vi "Check Channel Technique Compatibility.vi"(8 "error in (no error)":errorcluster, 9 "Technique in":T1, 10 "Channel":u8, 11 "Potentiostat Galvanostat in":refnum<class "Potentiostat Galvanostat.lvclass">) -> (0 "error out":errorcluster, 1 "Technique out":T1, 2 "Is Comapatible?":bool, 3 "Potentiostat Galvanostat out":refnum<class "Potentiostat Galvanostat.lvclass">)   [LabVIEW 2018, in "Potentiostat Galvanostat.lvclass"]
uses:
  Potentiostat Galvanostat.lvclass
  Controls/Technique List.ctl
  Controls/Error Codes.ctl
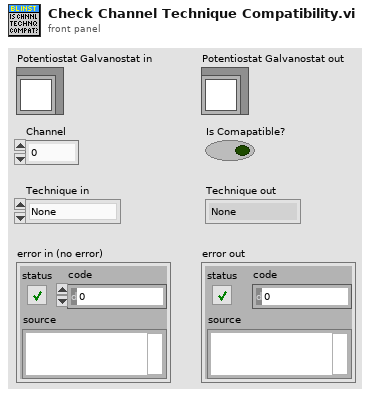
[diagram p1: front panel]
types:
  T1 = typedef "Potentiostat Galvanostat.lvclass/Technique List.ctl" = enum16{"None", "ocv", "cv", "biovscan", "ca", "cp", "iscan", "vscan", "lasv", "load", "pow", "peis", "geis", "seisp", "seisg", "dpv", "swv", "npv", "mpv", "dnpv", "dpa", "evt", "lp", "gc", "cpp", "pdp", "psp", "zra", "ircmp", "pzir", "gzir", "loop", "TO", "TI", "TOS", "vscanlimit", "iscanlimit", "mp", "casp", "casg", "calimit", "cplimit"}
  T2 = typedef "Potentiostat Galvanostat.lvclass/Error Codes.ctl" = i32
  T3 = typedef "Potentiostat Galvanostat.lvclass/Channel Information.ctl" = cluster{"Channel":i32, "Board Version":i32, "Board Serial Number":i32, "Firmware Code":T4, "Firmware Version":i32, "Xilinx Version":i32, "Amplifier Code":T5, "Number of Amplifiers":i32, "Low Current Board Present?":i32, "Impedance Capable?":i32, "RESERVED":i32, "RESERVED 2":i32, "Memory Size":i32, "Memory Filled (in Bytes)":i32, "Channel State":T6, "Maximum Current Range Allowed":T7, "Minimum Current Range Allowed":T7, "Maximum Bandwidth":T8, "Number of Techniques":i32}
  T4 = typedef "Potentiostat Galvanostat.lvclass/Firmware Code.ctl" = i32
  T5 = typedef "Potentiostat Galvanostat.lvclass/Amplifier Type.ctl" = i32
  T6 = typedef "Potentiostat Galvanostat.lvclass/Channel State.ctl" = i32
  T7 = typedef "Potentiostat Galvanostat.lvclass/Current Range.ctl" = i32
  T8 = typedef "Potentiostat Galvanostat.lvclass/Bandwidth.ctl" = i32
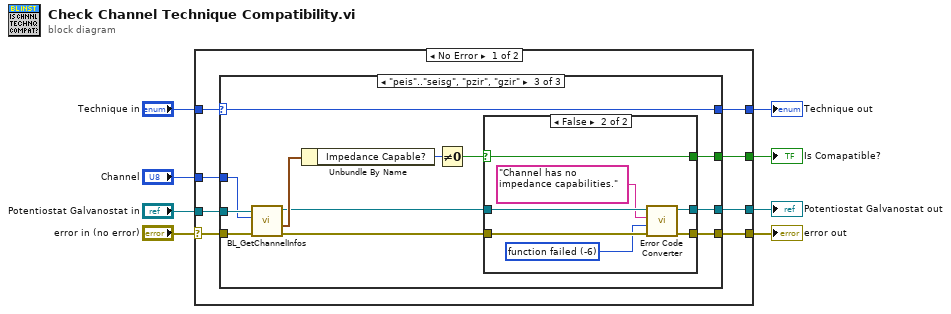
[diagram p0: block diagram]
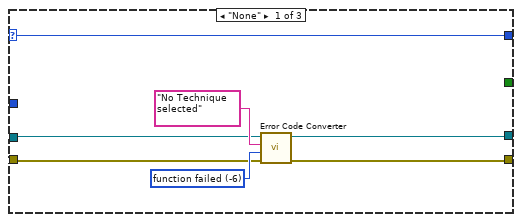
[diagram p2: hidden frame]
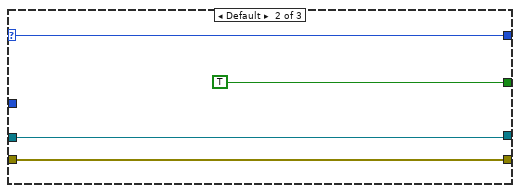
[diagram p3: hidden frame]
diagram:
  n1 = case shown="No Error" "error in (no error)" {
    selector: "error in (no error)" -> [w9 w50]
    tunnel: [w16 _] -> w8
    tunnel: [w15 w50] -> w7
    tunnel: [w14 w52] -> w6
    tunnel: [w13 w51] -> w5
    tunnel: "Channel" -> [w12 _]
    tunnel: "Potentiostat Galvanostat in" -> [w11 w52]
    tunnel: "Technique in" -> [w10 w51]
    frame No Error {
      n2 = case shown="\"peis\"..\"seisg\", \"pzir\", \"gzir\"" w10 {
        selector: w10 -> [w17 w25 w29]
        tunnel: w11 -> [w21 w27 w34]
        tunnel: w9 -> [w20 w26 w33]
        tunnel: w12 -> [_ _ w32]
        tunnel: [w18 w27 w31] -> w14
        tunnel: [w19 w26 w30] -> w15
        tunnel: [w17 w25 w29] -> w13
        tunnel: [_ TRUE w28] -> w16
        frame "None" {
          w23 = T2 -6 items=["No Error"=0, "no instrument connected"=-1, "connection in progress"=-2, "selected channel(s) unplugged"=-3, "invalid function parameters"=-4, "selected file does not exist"=-5, "function failed"=-6, "no channel selected"=-7, "invalid instrument configuration"=-8, "EC-Lab firmware loaded on the instrument"=-9, "library not correctly loaded in memory"=-10, "USB library not correctly loaded in memory"=-11, "function of the library already in progress"=-12, "selected channel(s) already used"=-13, "device not allowed"=-14, "Invalid update function parameters"=-15, "internal instrument communication failed"=-101, "too many data to transfer from the instrument (device error)"=-102, "selected channel(s) unplugged (device error)"=-103, "instrument response error"=-104, "invalid message size"=-105] ("Error Code")
          n3 = call-dynamic "Error Code Converter.vi"("error in (no error)"=w20, "Error Code"=w23, "Additional Description"="No Technique selected" ("error source (\" \")"), "Potentiostat Galvanostat in"=w21) -> ("error out"=w19:errorcluster, "Potentiostat Galvanostat out"=w18:refnum<class "Potentiostat Galvanostat.lvclass">)  [unwired: 6 in]
        }
        frame Default {
        }
        frame "peis".."seisg", "pzir", "gzir" {
          n4 = call-dynamic "BL_GetChannelInfos.vi"("error in (no error)"=w33, "Channel"=w32, "Potentiostat Galvanostat in"=w34) -> ("error out"=w36:errorcluster, "Channel Information"=w38:T3, "Potentiostat Galvanostat out"=w35:refnum<class "Potentiostat Galvanostat.lvclass">)  [unwired: 5 in, 1 out]
          n5 = Unbundle By Name(w38) -> ("Impedance Capable?"=w37:i32)
          n6 = Not Equal To 0?(x=w37) -> (x != 0?=w39:bool)
          n7 = case shown="False" w39 {
            selector: w39 -> [w40 w43]
            tunnel: w36 -> [w41 w49]
            tunnel: w35 -> [w42 w48]
            tunnel: [w42 w45] -> w31
            tunnel: [w41 w44] -> w30
            tunnel: [w40 w43] -> w28
            frame True {
            }
            frame False {
              w47 = T2 -6 items=["No Error"=0, "no instrument connected"=-1, "connection in progress"=-2, "selected channel(s) unplugged"=-3, "invalid function parameters"=-4, "selected file does not exist"=-5, "function failed"=-6, "no channel selected"=-7, "invalid instrument configuration"=-8, "EC-Lab firmware loaded on the instrument"=-9, "library not correctly loaded in memory"=-10, "USB library not correctly loaded in memory"=-11, "function of the library already in progress"=-12, "selected channel(s) already used"=-13, "device not allowed"=-14, "Invalid update function parameters"=-15, "internal instrument communication failed"=-101, "too many data to transfer from the instrument (device error)"=-102, "selected channel(s) unplugged (device error)"=-103, "instrument response error"=-104, "invalid message size"=-105] ("Error Code")
              n8 = call-dynamic "Error Code Converter.vi"("error in (no error)"=w49, "Error Code"=w47, "Additional Description"="Channel has no impedance capabilities." ("error source (\" \")"), "Potentiostat Galvanostat in"=w48) -> ("error out"=w44:errorcluster, "Potentiostat Galvanostat out"=w45:refnum<class "Potentiostat Galvanostat.lvclass">)  [unwired: 6 in]
            }
          }
        }
      }
    }
    frame Error {
    }
  }
  "Is Comapatible?" <- w8
  "error out" <- w7
  "Potentiostat Galvanostat out" <- w6
  "Technique out" <- w5
